vi "niDTS GNSS Dut Close.vi"(0 "GNSS Dut Handle in":T2, 11 "error in (no error)":errorcluster, 13 "Force Destroy? (F)":T1) -> (15 "error out":errorcluster)   [LabVIEW 2014, in "niDTS GNSS.lvlib"]
uses:
  niDTS GNSS.lvlib
  Includes/niDTS GNSS Dut INC Handle.ctl
  Objects/BASE_class/niDTS GNSS Dut.lvclass
  Framework/Session/Includes/niDTS Session INC Force Destroy.ctl
  Framework/niDTS Framework.lvlib
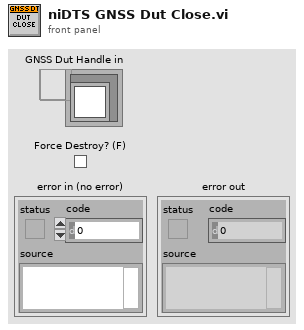
[diagram p1: front panel]
types:
  T1 = typedef "niDTS Framework.lvlib/niDTS Session INC Force Destroy.ctl" = bool
  T2 = typedef "niDTS GNSS.lvlib/niDTS GNSS Dut INC Handle.ctl" = refnum<data-value>
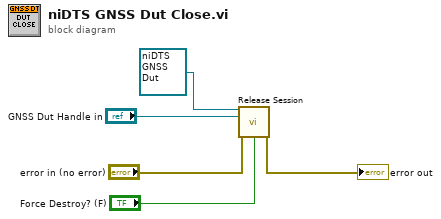
[diagram p0: block diagram]
diagram:
  n1 = call-dynamic "Release Session.vi"("OBJ - Session in"=refnum<class "niDTS GNSS Dut.lvclass"> refnum ("niDTS GPS.lvlib:Template Dut"), "Session Handle in"="GNSS Dut Handle in", "error in (no error)"="error in (no error)", "Force Destroy? (F)"="Force Destroy? (F)") -> ("error out"=→"error out":errorcluster)  [unwired: 10 in, 1 out]
